vi "Enqueue Message.vi"   [LabVIEW 2016, in "Message Queue.lvlib"]
uses:
  Message Queue.lvlib
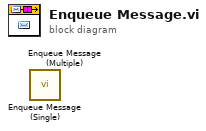
[diagram p0: block diagram]
diagram:
  n1 = call "Enqueue Message (Single).vi"() -> ()  [unwired: 10 in, 2 out]
  n2 = call "Enqueue Message (Multiple).vi"() -> ()  [unwired: 10 in, 2 out]
